vi "Is Pre Amp Gain Available.vi"(6 "status":i32, 7 "pa":i32, 9 "index":i32, 10 "amplifier":i32, 11 "channel":i32) -> (3 "function return":u32, 4 "status out":i32)   [LabVIEW 2018, in "Copy of Andor SDK.lvlib"]
doc: "EXPNETTYPE unsigned int WINAPI IsPreAmpGainAvailable(int channel, int amplifier, int index, int pa, int * status);"
uses:
  Copy of Andor SDK.lvlib
  <userlib>/Andor SDK/ATMCD32D.dll
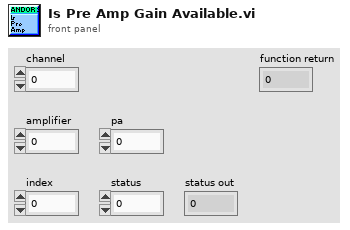
[diagram p1: front panel]
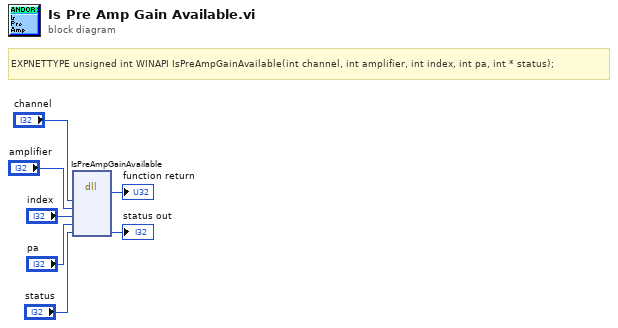
[diagram p0: block diagram]
diagram:
  # "EXPNETTYPE unsigned int WINAPI IsPreAmpGainAvailable(int channel, int amplifier, int index, int pa, int * status);"
  n1 = dll-call lib="C:/Program Files (x86)/National Instruments/LabVIEW 2018/user.lib/Andor SDK/ATMCD32D.*" fn="IsPreAmpGainAvailable"("channel"="channel", "amplifier"="amplifier", "index"="index", "pa"="pa", "status"="status") -> (→"function return":u32, "status"=→"status out":i32)  [unwired: 7 in, 2 out]
